vi "G#InterfaceImplementation_Create.vi"(0 "reference in":refnum<class "G#Object.lvclass">, 5 "error in (no error)":errorcluster) -> (14 "reference out":refnum<class "G#InterfaceImplementation.lvclass">, 19 "error out":errorcluster)   [LabVIEW 2017, in "G#InterfaceImplementation.lvclass"]
doc: "Creates the interface for the G#Object."
uses:
  <vilib>/addons/_AddQ/G#Templates/G#InterfaceImplementation/G#InterfaceImplementation.lvclass
  C:/Program Files (x86)/National Instruments/LabVIEW 2017/vi.lib/addons/_AddQ/G#Templates/G#InterfaceTemplate/G#InterfaceTemplate.lvclass
  <vilib>/addons/_AddQ/G#Object/G#Object.lvclass
  <vilib>/addons/_AddQ/G#Templates/G#InterfaceTemplate/G#InterfaceTemplate.lvclass
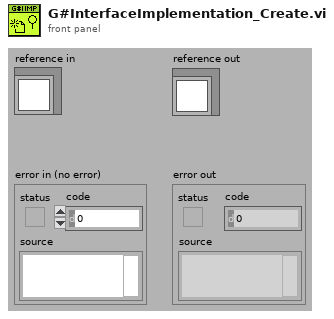
[diagram p1: front panel]
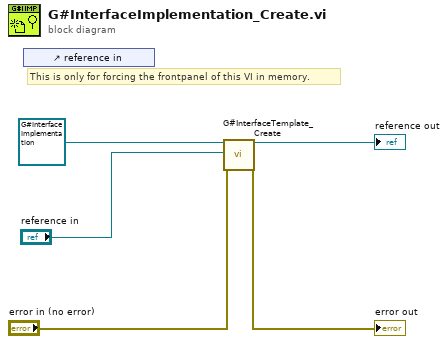
[diagram p0: block diagram]
diagram:
  # "This is only for forcing the frontpanel of this VI in memory."
  n1 = control-ref of="reference in"() -> ()  [unwired: 1 out]
  n2 = call <vilib>:"G#InterfaceTemplate_Create.vi"("reference in"=refnum<class "G#InterfaceImplementation.lvclass"> refnum ("reference out"), "G#Object in"="reference in", "error in (no error)"="error in (no error)") -> ("reference out"=→"reference out":refnum<class "G#InterfaceImplementation.lvclass">, "error out"=→"error out":errorcluster)  [unwired: 15 in]
